vi "Handle.vi"(11 "jettl in":refnum<class "jettl.lvclass">) -> (3 "jettl out":refnum<class "jettl.lvclass">)   [LabVIEW 2021, in "jettl.lvlib" / "jettl.lvclass"]
uses:
  jettl.lvclass
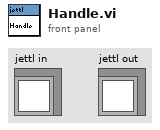
[diagram p1: front panel]
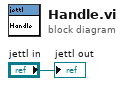
[diagram p0: block diagram]
diagram:
  "jettl out" <- "jettl in"
